vi "Main NR.vi"(8 "error in":errorcluster, 11 "Head Worker in":refnum<class "Head Worker.lvclass">) -> (0 "error out":errorcluster, 3 "Head Worker out":refnum<class "Head Worker.lvclass">)   [LabVIEW 2017, in "Head Worker.lvclass"]
doc: "The <b>Queued Message Handler</b> of the Worker that owns this VI."
uses:
  Head Worker.lvclass
  C:/Program Files (x86)/National Instruments/LabVIEW 2017/vi.lib/addons/_Workers/Library/Classes/Worker/Worker.lvclass
  Head Worker.lvclass/Head Worker.ctl
  Initialization Data.ctl
  TCP Client/TCP Client/rwr_Connect to Server.ctl
  TCP Client/TCP Client/rqp_Send String to Server.ctl
  TCP Client/TCP Client/TCP Client.lvclass
panel:
  out "IP Address":string caption="Server IP Address"
  out "Server name":string caption="Server Name"
  out "String Received from Server":string
  out "Connected?":bool
  # "Server Connected"
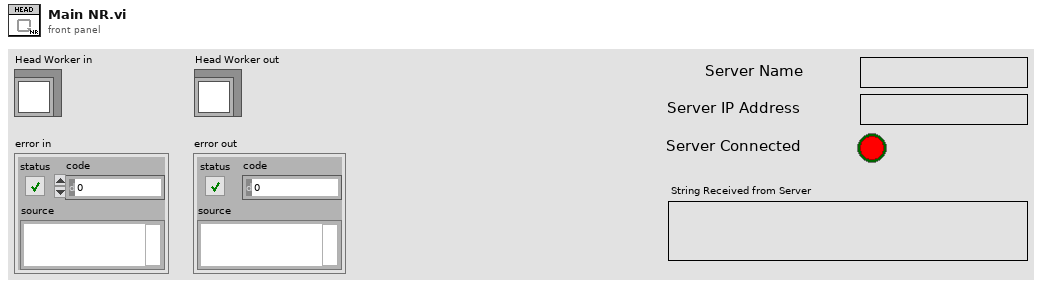
[diagram p1: front panel]
types:
  T1 = typedef "Head Worker.lvclass/Initialization Data.ctl" = cluster{"Client Name":string, "Server IP Address":string, "Server Port":u16}
  T2 = typedef "TCP Client.lvlib/TCP Client.lvclass/rwr_Connect to Server.ctl" = cluster{"Client Name":string, "Server IP Address":string, "Server Port":u16}
  T3 = typedef "TCP Client.lvlib/TCP Client.lvclass/rqp_Send String to Server.ctl" = cluster{"String to Send":string}
  T4 = typedef "TCP Client.lvlib/TCP Client.lvclass/rsp_Connection Notify.ctl" = cluster{"Server Name":string, "IP Address":string, "Connected?":bool}
  T5 = typedef "TCP Client.lvlib/TCP Client.lvclass/rsp_Incoming Data.ctl" = cluster{"Data":string}
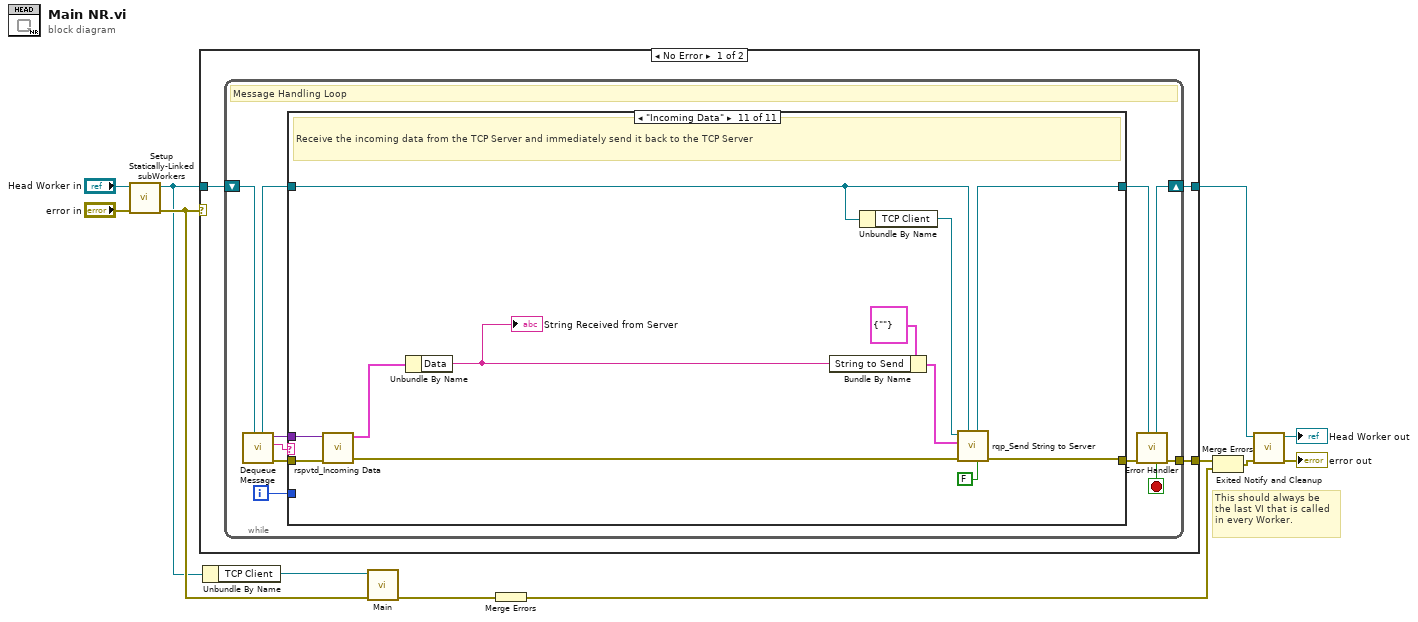
[diagram p0: block diagram]
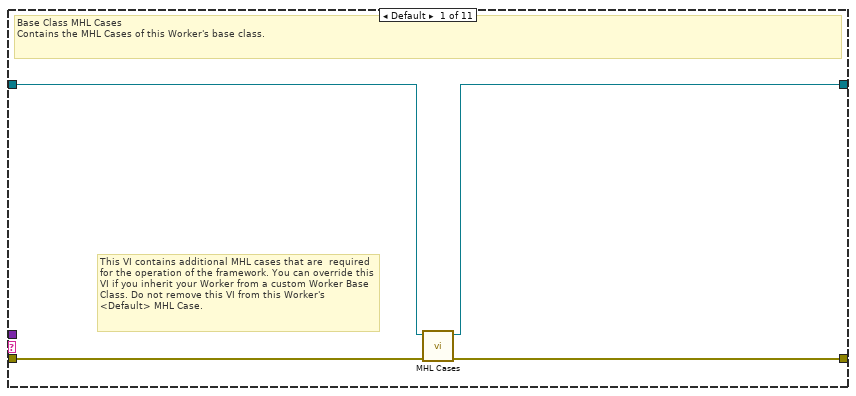
[diagram p2: hidden frame]
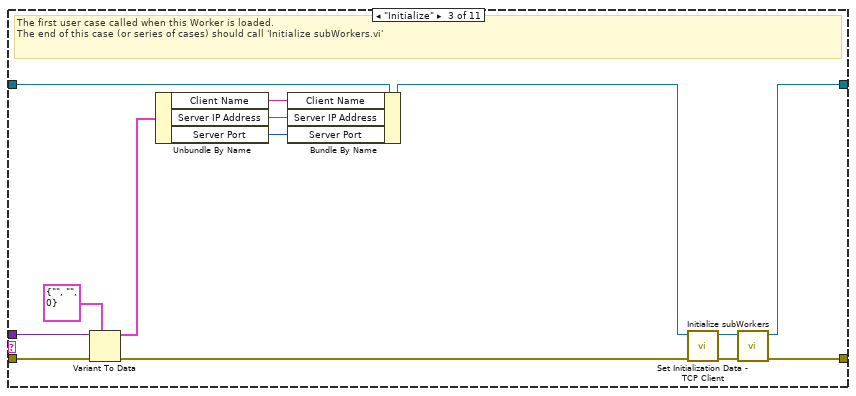
[diagram p4: hidden frame]
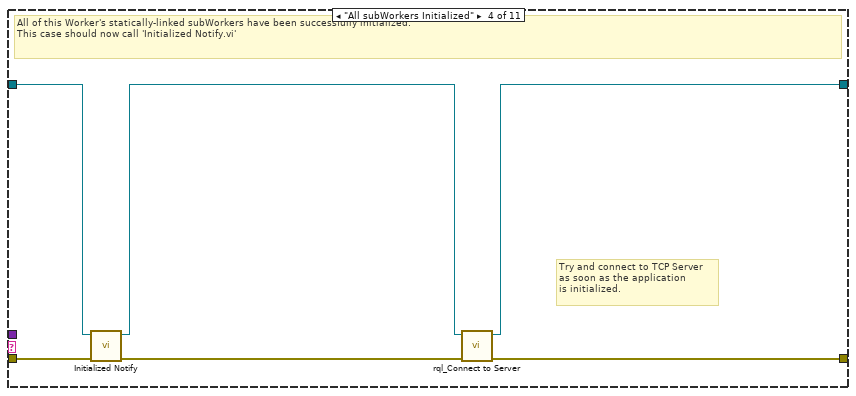
[diagram p5: hidden frame]
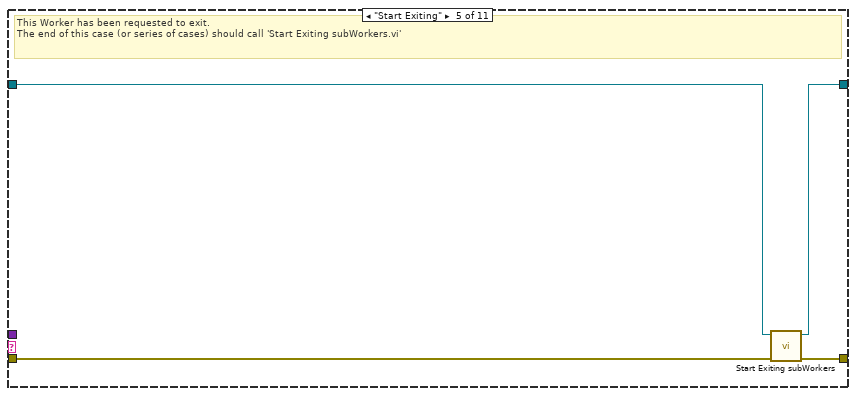
[diagram p6: hidden frame]
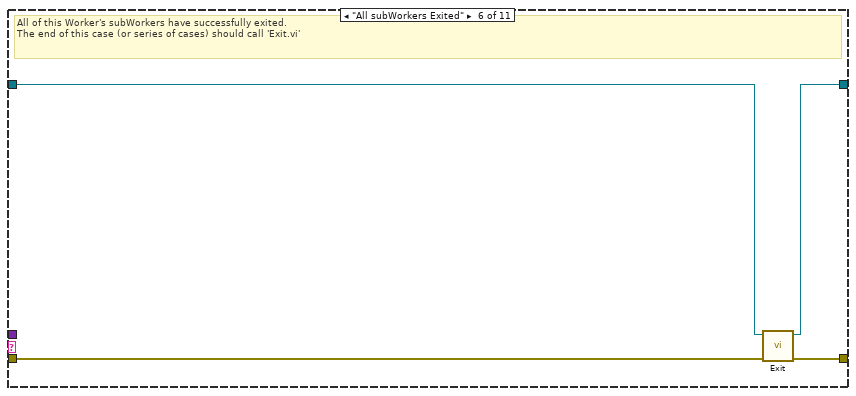
[diagram p7: hidden frame]
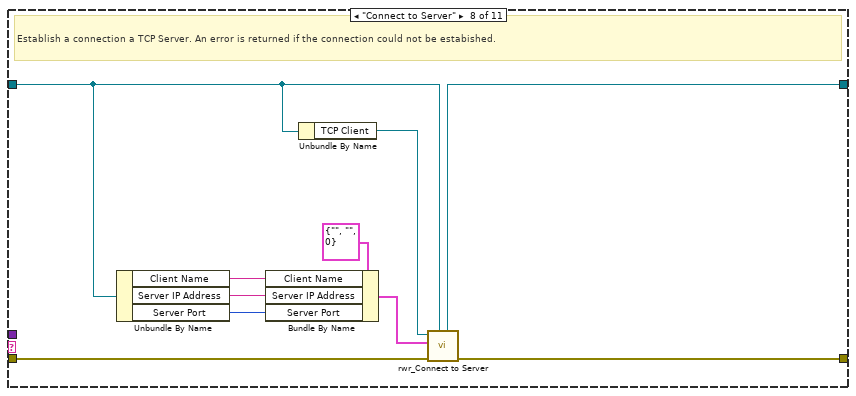
[diagram p9: hidden frame]
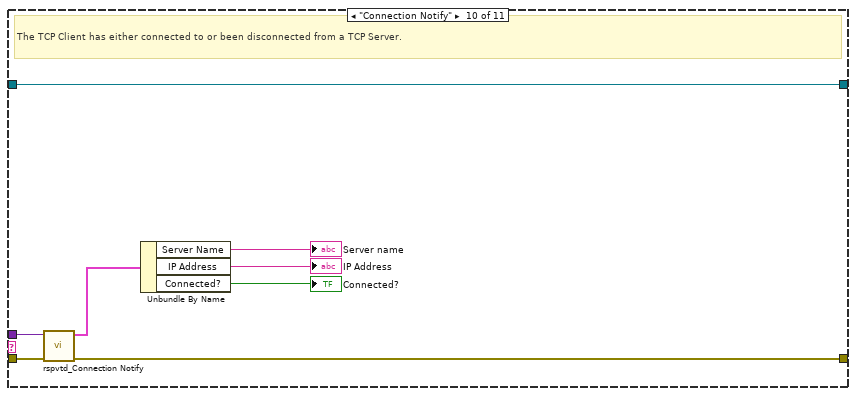
[diagram p11: hidden frame]
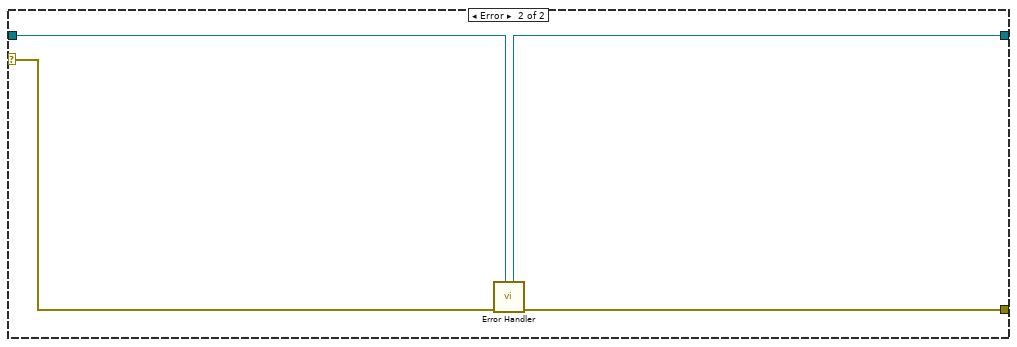
[diagram p12: hidden frame]
diagram:
  # "This should always be the last VI that is called in every Worker."
  n1 = call "Setup Statically-Linked subWorkers.vi"("error in"="error in", "Head Worker in"="Head Worker in") -> ("error out"=w6:errorcluster, "Head Worker out"=w4:refnum<class "Head Worker.lvclass">)  [unwired: 8 in]
  n2 = case shown="No Error" w6 {
    tunnel: w4 -> [w15 w96]
    tunnel: [w13 w97] -> w10
    tunnel: [w14 w95] -> w11
    selector: w6 -> [_ w98]
    frame No Error {
      n3 = while {
        shift-right: [w24] -> w14
        shift-left: w15 -> [w26]
        tunnel: [w25] -> w13
        i -> [w17]
        stop <- w18 stop-if-true
        # "Message Handling Loop"
        n4 = call-dynamic "Dequeue Message.vi"("Worker"=w26) -> ("error out"=w23:errorcluster, "Case out"=w19:string, "Data out"=w16:variant, "Worker out"=w21:refnum<class "Head Worker.lvclass">)  [unwired: 6 in, 1 out]
        n5 = case "Worker MHL Case Structure (DO NOT CHANGE LABEL NAME)" shown="\"Incoming Data\"" w19 {
          tunnel: w23 -> [w30 w31 w44 w51 w53 w60 w62 w72 w74 w82 w94]
          tunnel: [w29 w31 w46 w50 w56 w59 w62 w71 w74 w80 w83] -> w22
          tunnel: w21 -> [w28 w32 w37 w52 w54 w58 w61 w66 w73 w81 w86]
          tunnel: [w27 w32 w45 w49 w55 w57 w61 w70 w73 w81 w87] -> w20
          tunnel: w17 -> [_ _ _ _ _ _ _ _ _ _ _]
          tunnel: w16 -> [_ _ w42 _ _ _ _ _ _ w79 w93]
          frame Default {
            # "This VI contains additional MHL cases that are  required for the operation of the framework. You can override this VI if you inherit your Worker from a custom Worker Base Class. Do not remove this VI from this Worker's <Default> MHL Case."
            # "Base Class MHL Cases\nContains the MHL Cases of this Worker's base class."
            n6 = call-dynamic "MHL Cases.vi"("error in"=w30, "Worker in"=w28) -> ("error out"=w29:errorcluster, "Worker out"=w27:refnum<class "Head Worker.lvclass">)  [unwired: 8 in]
          }
          frame "------------ FRAMEWORK CASES -----------" {
            # "Start of Workers Framework Cases"
          }
          frame "Initialize" {
            # "The first user case called when this Worker is loaded.\nThe end of this case (or series of cases) should call 'Initialize subWorkers.vi'"
            n7 = Variant To Data(error in=w44, type=T1 {"Client Name"="", "Server IP Address"="", "Server Port"=0} ("Initialization Data"), Variant=w42) -> (data=w40:T1, error out=w43:errorcluster)
            n8 = Unbundle By Name(w40) -> ("Client Name"=w35:string, "Server IP Address"=w34:string, "Server Port"=w33:u16)
            n9 = Bundle By Name(cluster=w37, "Client Name"=w35, "Server IP Address"=w34, "Server Port"=w33) -> (w36:refnum<class "Head Worker.lvclass">)
            n10 = call "Set Initialization Data - TCP Client.vi"("error in"=w43, "Head Worker in"=w36) -> ("error out"=w39:errorcluster, "Head Worker out"=w38:refnum<class "Head Worker.lvclass">)  [unwired: 8 in]
            n11 = call-dynamic "Initialize subWorkers.vi"("error in"=w39, "Worker"=w38) -> ("error out"=w46:errorcluster, "dup Worker out"=w45:refnum<class "Head Worker.lvclass">)  [unwired: 8 in]
          }
          frame "All subWorkers Initialized" {
            # "Try and connect to TCP Server\nas soon as the application\nis initialized."
            # "All of this Worker's statically-linked subWorkers have been successfully initialized.\nThis case should now call 'Initialized Notify.vi'"
            n12 = call-dynamic "Initialized Notify.vi"("error in"=w51, "Worker"=w52) -> ("error out"=w47:errorcluster, "dup Worker out"=w48:refnum<class "Head Worker.lvclass">)  [unwired: 8 in]
            n13 = call "rql_Connect to Server.vi"("error in"=w47, "Head Worker in"=w48) -> ("error out"=w50:errorcluster, "dup Head Worker out"=w49:refnum<class "Head Worker.lvclass">)  [unwired: 8 in]
          }
          frame "Start Exiting" {
            # "This Worker has been requested to exit. \nThe end of this case (or series of cases) should call 'Start Exiting subWorkers.vi'"
            n14 = call-dynamic "Start Exiting subWorkers.vi"("error_in"=w53, "Worker"=w54) -> ("error out"=w56:errorcluster, "dup Worker out"=w55:refnum<class "Head Worker.lvclass">)  [unwired: 8 in]
          }
          frame "All subWorkers Exited" {
            # "All of this Worker's subWorkers have successfully exited. \nThe end of this case (or series of cases) should call 'Exit.vi'"
            n15 = call-dynamic "Exit.vi"("error_in"=w60, "Worker"=w58) -> ("error out"=w59:errorcluster, "dup Worker out"=w57:refnum<class "Head Worker.lvclass">)  [unwired: 8 in]
          }
          frame "------------- LOCAL API CASES -------------" {
            # "Start of Workers Local API Cases"
          }
          frame "Connect to Server" {
            # "Establish a connection a TCP Server. An error is returned if the connection could not be estabished."
            n16 = Unbundle By Name(w66) -> ("Client Name"=w65:string, "Server IP Address"=w64:string, "Server Port"=w63:u16)
            n17 = Bundle By Name(cluster=T2 {"Client Name"="", "Server IP Address"="", "Server Port"=0} ("Connect to Server Data"), "Client Name"=w65, "Server IP Address"=w64, "Server Port"=w63) -> (w68:T2)
            n18 = Unbundle By Name(w66) -> ("TCP Client"=w67:refnum<class "TCP Client.lvclass">)
            n19 = call "rwr_Connect to Server.vi"("Caller in"=w66, "error in"=w72, "Data in"=w68, "TCP Client in"=w67) -> ("error out"=w71:errorcluster, "dup Caller out"=w70:refnum<class "Head Worker.lvclass">)  [unwired: 4 in, 2 out]
          }
          frame "------------- RESPONSE CASES --------------" {
            # "Start of Workers Response Cases"
          }
          frame "Connection Notify" {
            # "The TCP Client has either connected to or been disconnected from a TCP Server."
            n20 = call "rspvtd_Connection Notify.vi"("error in"=w82, "Data in"=w79) -> ("error out"=w80:errorcluster, "Data out"=w76:T4)  [unwired: 8 in]
            n21 = Unbundle By Name(w76) -> ("Server Name"=→"Server name":string, "IP Address"=→"IP Address":string, "Connected?"=→"Connected?":bool)
          }
          frame "Incoming Data" {
            # "Receive the incoming data from the TCP Server and immediately send it back to the TCP Server"
            n22 = call "rspvtd_Incoming Data.vi"("error in"=w94, "Data in"=w93) -> ("error out"=w84:errorcluster, "Data out"=w92:T5)  [unwired: 8 in]
            n23 = Unbundle By Name(w92) -> ("Data"=w88:string)
            "String Received from Server" <- w88
            n24 = Bundle By Name(cluster=T3 {"String to Send"=""} ("Data in"), "String to Send"=w88) -> (w90:T3)
            n25 = Unbundle By Name(w86) -> ("TCP Client"=w85:refnum<class "TCP Client.lvclass">)
            n26 = call "rqp_Send String to Server.vi"("Show in Debugger?"=FALSE, "Caller in"=w86, "error in"=w84, "Data in"=w90, "TCP Client in"=w85) -> ("error out"=w83:errorcluster, "dup Caller out"=w87:refnum<class "Head Worker.lvclass">)  [unwired: 4 in, 1 out]
          }
        }
        n27 = call-dynamic "Error Handler.vi"("Worker"=w20, "error_in"=w22) -> ("error out"=w25:errorcluster, "Stop Loop"=w18:bool, "Worker out"=w24:refnum<class "Head Worker.lvclass">)  [unwired: 7 in]
      }
    }
    frame Error {
      n28 = call-dynamic "Error Handler.vi"("Worker"=w96, "error_in"=w98) -> ("error out"=w97:errorcluster, "Worker out"=w95:refnum<class "Head Worker.lvclass">)  [unwired: 7 in, 1 out]
    }
  }
  n29 = Unbundle By Name(w4) -> ("TCP Client"=w1:refnum<class "TCP Client.lvclass">)
  n30 = call-dynamic "Main.vi"("error in"=w6, "TCP Client in"=w1) -> ("error out"=w3:errorcluster)  [unwired: 8 in, 1 out]
  n31 = Merge Errors(w3) -> (w2:errorcluster)
  n32 = Merge Errors(w10, w2) -> (w12:errorcluster)
  n33 = call-dynamic "Exited Notify and Cleanup.vi"("error_in"=w12, "Worker"=w11) -> ("error out"=→"error out":errorcluster, "dup Worker out"=→"Head Worker out":refnum<class "Head Worker.lvclass">)  [unwired: 8 in]
